vi "Voltage_to_Thrust.vi"(2 "Right Voltage":dbl[](array[numeric]) format="%_6g", 3 "Left Voltage":dbl[](array[numeric]) format="%_6g") -> (0 "Right Thrust":dbl[](array[numeric]) format="%_6g", 1 "Left Thrust":dbl[](array[numeric]) format="%_6g")   [LabVIEW 2009]
uses:
  <vilib>/gmath/NI_Gmath.lvlib
panel:
  in  "Right Voltage / Thrust":cluster{"V":dbl, "T":dbl}[](array[cluster])
  in  "Left Voltage / Thrust":cluster{"V":dbl, "T":dbl}[](array[cluster])
  # "Voltage is in V\nThrust in N"
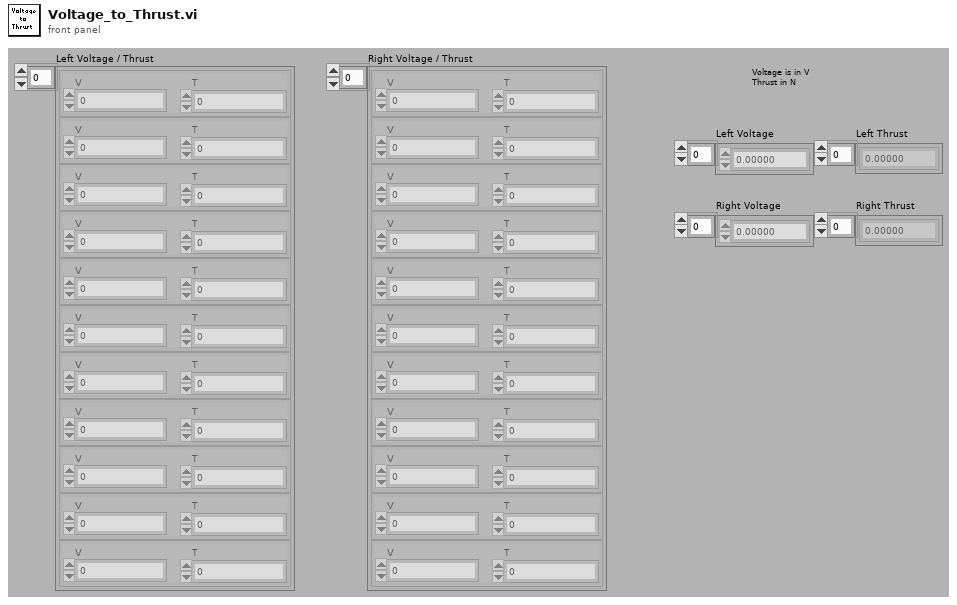
[diagram p1: front panel]
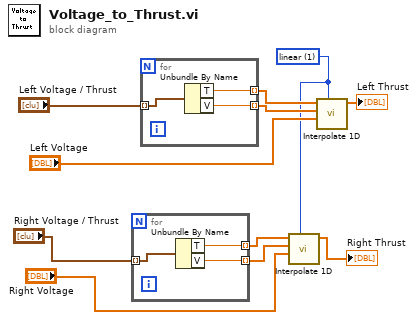
[diagram p0: block diagram]
diagram:
  w5 = 1 items=["nearest", "linear", "spline", "cubic Hermite", "Lagrange"] ("method")
  n1 = for {
    tunnel: "Right Voltage / Thrust" -> [w14] mode=indexing
    tunnel: [w13] -> w3 mode=indexing
    tunnel: [w12] -> w2 mode=indexing
    n2 = Unbundle By Name(w14) -> ("T"=w13:dbl, "V"=w12:dbl)
  }
  n3 = for {
    tunnel: "Left Voltage / Thrust" -> [w17] mode=indexing
    tunnel: [w16] -> w10 mode=indexing
    tunnel: [w15] -> w9 mode=indexing
    n4 = Unbundle By Name(w17) -> ("T"=w16:dbl, "V"=w15:dbl)
  }
  n5 = call <vilib>:"Interpolate 1D.vi"("method"=w5, "xi"="Right Voltage", "X"=w2, "Y"=w3) -> ("yi"=→"Right Thrust":dbl[])  [unwired: 5 in, 2 out]
  n6 = call <vilib>:"Interpolate 1D.vi"("method"=w5, "xi"="Left Voltage", "X"=w9, "Y"=w10) -> ("yi"=→"Left Thrust":dbl[])  [unwired: 5 in, 2 out]
